vi "Configure Pseudocard.vi"(0 "VISA resource name":refnum<visa-resource-name>, 5 "Slot Number (1)":i32=1, 9 "Pseudocard Name (0: C7700)":u16(ring) items=["C7700", "C7701", "C7702", "C7703", "C7705", "C7706", "C7707", "C7708", "C7709"], 11 "error in (no error)":errorcluster) -> (4 "VISA resource name out":refnum<visa-resource-name>, 15 "error out":errorcluster)   [LabVIEW 2020, in "Keithley 27XX.lvlib"]
doc: "This VI installs a pseudocard into the DMM. A pseudocard is a virtual card which can be helpful when designing applications which use particular cards."
uses:
  Keithley 27XX.lvlib
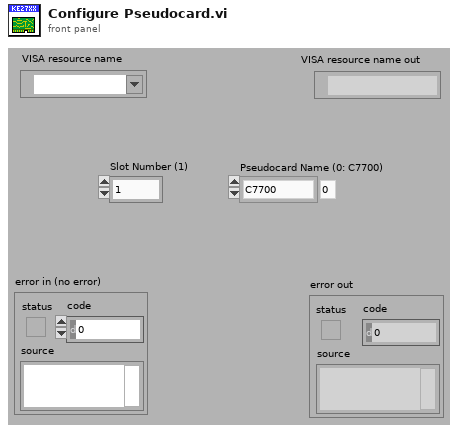
[diagram p1: front panel]
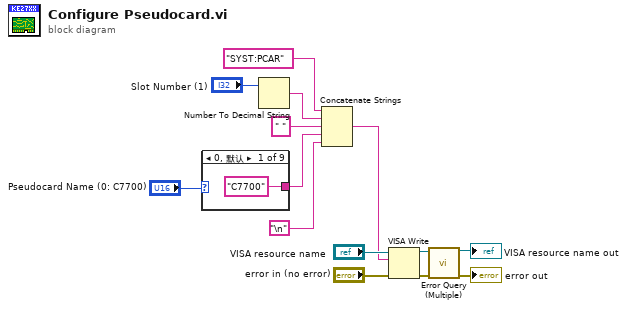
[diagram p0: block diagram]
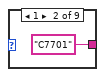
[diagram p2: hidden frame]
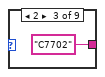
[diagram p3: hidden frame]
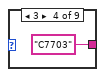
[diagram p4: hidden frame]
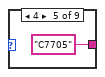
[diagram p5: hidden frame]
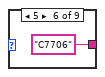
[diagram p6: hidden frame]
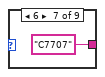
[diagram p7: hidden frame]
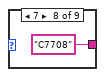
[diagram p8: hidden frame]
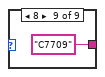
[diagram p9: hidden frame]
diagram:
  n1 = case shown="0, 默认" "Pseudocard Name (0: C7700)" {
    tunnel: ["C7700" "C7701" "C7702" "C7703" "C7705" "C7706" "C7707" "C7708" "C7709"] -> w9
    frame 0, Default {
    }
    frame 1 {
    }
    frame 2 {
    }
    frame 3 {
    }
    frame 4 {
    }
    frame 5 {
    }
    frame 6 {
    }
    frame 7 {
    }
    frame 8 {
    }
  }
  n2 = Number To Decimal String(number="Slot Number (1)") -> (decimal integer string=w11:string)  [unwired: 1 in]
  n3 = Concatenate Strings("SYST:PCAR", w11, " ", w9, "\n") -> (w6:string)
  n4 = VISA Write(VISA resource name="VISA resource name", write buffer=w6, error in (no error)="error in (no error)") -> (VISA resource name out=w5:refnum<visa-resource-name>, error out=w4:errorcluster)  [unwired: 1 out]
  n5 = call "Error Query (Multiple).vi"("VISA resource name"=w5, "error in (no error)"=w4) -> ("VISA resource name out"=→"VISA resource name out":refnum<visa-resource-name>, "error out"=→"error out":errorcluster)  [unwired: 10 in, 2 out]
